vi "process.vi"(8 "error in":errorcluster, 9 "result allocation":T1, 10 "parameters":T1, 11 "module in":refnum<class "Sequencer Module runtime.lvclass">) -> (0 "error out":errorcluster, 1 "results":T1, 2 "parameter allocation":T1, 3 "module out":refnum<class "Sequencer Module runtime.lvclass">)   [LabVIEW 2015, in "Sequencer Module runtime.lvclass"]
doc: "Provides an interface for information processing by a module at runtime. While this interface performs no operations, a child should provide an override which may process data in any manner necessary."
uses:
  Sequencer Module runtime.lvclass
  <vilib>/NI/Tag Bus/table/data table.ctl
  Sequencer Module runtime.lvclass/Sequencer Module runtime.ctl
  classes/Sequence/Sequence.lvclass
  classes/Step/Step.lvclass
  <vilib>/NI/Tag Bus/table/data table.lvlib
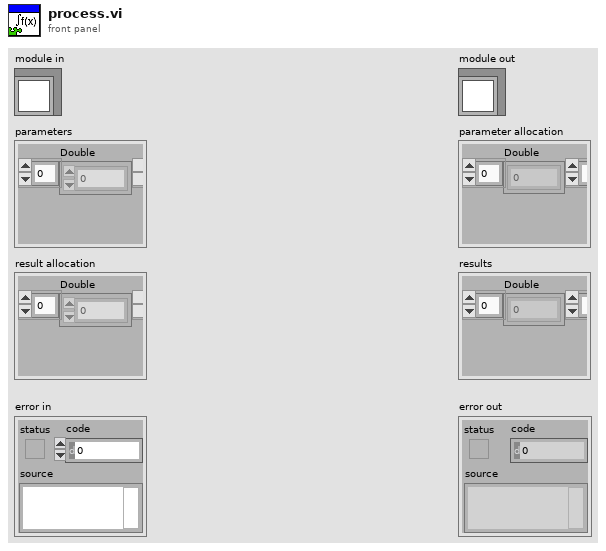
[diagram p1: front panel]
types:
  T1 = typedef "tag bus.lvlib/data table.lvlib/data table.ctl" = cluster{"Double":dbl[], "Single":sgl[], "I64":i64[], "I32":i32[], "I16":i16[], "I8":i8[], "U64":u64[], "U32":u32[], "U16":u16[], "U8":u8[], "Boolean":bool[], "String":string[], "Array of Double":cluster{"DBL Array":dbl[]}[], "Array of Single":cluster{"SGL Array":sgl[]}[], "Array of I64":cluster{"I64 Array":i64[]}[], "Array of I32":cluster{"I32 Array":i32[]}[], "Array of I16":cluster{"I16 Array":i16[]}[], "Array of I8":cluster{"I8 Array":i8[]}[], "Array of U64":cluster{"U64 Array":u64[]}[], "Array of U32":cluster{"U32 Array":u32[]}[], "Array of U16":cluster{"U16 Array":u16[]}[], "Array of U8":cluster{"U8 Array":u8[]}[], "Array of Boolean":cluster{"Boolean Array":bool[]}[], "Array of String":cluster{"String Array":string[]}[]}
  T2 = typedef "Sequencer Module configuration.lvclass/Sequencer State Enum.ctl" = enum16{"Running", "Paused"}
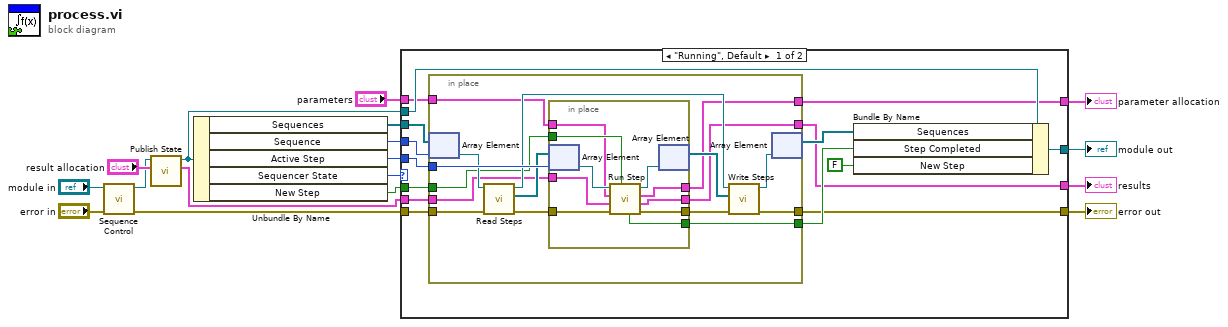
[diagram p0: block diagram]
diagram:
  n1 = call "Sequence Control.vi"("error in (no error)"="error in", "Sequencer Module runtime in"="module in") -> ("error out"=w9:errorcluster, "Sequencer Module runtime out"=w2:refnum<class "Sequencer Module runtime.lvclass">)  [unwired: 8 in]
  n2 = call "Publish State.vi"("result allocation in"="result allocation", "Sequencer Module runtime in"=w2) -> ("result allocation out"=w3:T1, "Sequencer Module runtime out"=w1:refnum<class "Sequencer Module runtime.lvclass">)  [unwired: 8 in]
  n3 = Unbundle By Name(w1) -> ("Sequences"=w16:refnum<class "Sequence.lvclass">[], "Sequence"=w15:i32, "Active Step"=w17:i32, "Sequencer State"=w12:T2, "New Step"=w8:bool)
  n4 = case shown="\"Running\", Default" w12 {
    tunnel: w17 -> [w32 _]
    tunnel: w16 -> [w31 _]
    tunnel: w15 -> [w30 _]
    tunnel: w9 -> [w29 w61]
    tunnel: w1 -> [w28 w62]
    tunnel: [w25 w62] -> w14
    tunnel: [w24 w61] -> w13
    tunnel: w8 -> [w23 _]
    tunnel: "parameters" -> [w21 w60]
    tunnel: [w20 w60] -> w6
    tunnel: w3 -> [w19 w59]
    tunnel: [w18 w59] -> w5
    frame "Running", Default {
      n5 = in-place {
        in-place-border: w32 -> [w48]
        in-place-border: w29 -> [w42]
        in-place-border: [w39] -> w24
        in-place-border: [w38] -> w26
        in-place-border: w23 -> [w37]
        in-place-border: w21 -> [w36]
        in-place-border: [w35] -> w20
        in-place-border: w19 -> [w34]
        in-place-border: [w33] -> w18
        n6 = in-place-array #1(w31, w30) -> (w47:refnum<class "Sequence.lvclass">)
        n7 = call-dynamic "Read Steps.vi"("error in (no error)"=w42, "Sequence in"=w47) -> ("error out"=w41:errorcluster, "Steps"=w46:refnum<class "Step.lvclass">[], "Sequence out"=w44:refnum<class "Sequence.lvclass">)  [unwired: 7 in]
        n8 = in-place {
          in-place-border: w41 -> [w56]
          in-place-border: [w55] -> w40
          in-place-border: [w53] -> w38
          in-place-border: w37 -> [w54]
          in-place-border: w36 -> [w52]
          in-place-border: [w51] -> w35
          in-place-border: w34 -> [w50]
          in-place-border: [w49] -> w33
          n9 = in-place-array #2(w46, w48) -> (w58:refnum<class "Step.lvclass">)
          n10 = call-dynamic "Run Step.vi"("New Step"=w54, "error in (no error)"=w56, "result allocation"=w50, "parameters"=w52, "Step in"=w58) -> ("error out"=w55:errorcluster, "results"=w49:T1, "parameter allocation"=w51:T1, "Step out"=w57:refnum<class "Step.lvclass">, "Completed"=w53:bool)  [unwired: 2 in]
          n11 = in-place-array #2(w57) -> (w45:refnum<class "Step.lvclass">[])  [unwired: 1 out]
        }
        n12 = call-dynamic "Write Steps.vi"("error in (no error)"=w40, "Steps"=w45, "Sequence in"=w44) -> ("error out"=w39:errorcluster, "Sequence out"=w43:refnum<class "Sequence.lvclass">)  [unwired: 7 in]
        n13 = in-place-array #1(w43) -> (w27:refnum<class "Sequence.lvclass">[])  [unwired: 1 out]
      }
      n14 = Bundle By Name(cluster=w28, "Sequences"=w27, "Step Completed"=w26, "New Step"=FALSE ("Sequencer State.New Step")) -> (w25:refnum<class "Sequencer Module runtime.lvclass">)
    }
    frame "Paused" {
    }
  }
  "module out" <- w14
  "results" <- w5
  "parameter allocation" <- w6
  "error out" <- w13
